vi "HGCalSensorTestingPanel2.vi"() -> ()   [LabVIEW 2015]
uses:
  <vilib>/Utility/file.llb/Write Delimited Spreadsheet (string).vi
panel:
  out "K237 count":u32
  in  "K237 VISA":refnum<visa-resource-name>
  out "XY Graph 2":cluster{"Y":dbl[], "Y":dbl[]}[](graph)
  out "return count 5":u32
  in  "write buffer 2":string
  out "return count 4":u32
  in  "VISA QT7600":refnum<visa-resource-name>
  in  "write buffer":string
  out "VISA out 3":refnum<visa-resource-name>
  out "return count 3":u32
  in  "byte count 2":u32
  out "XY Graph":cluster{"Y":dbl[], "Y":dbl[]}[](graph)
  out "VISA out 2":refnum<visa-resource-name>
  out "return count 2":u32
  out "error out 2":errorcluster
  in  "byte count":u32
  in  "HP":refnum<visa-resource-name>
  out "VISA out":refnum<visa-resource-name>
  out "return count":u32
  in  "Switch":refnum<visa-resource-name>
  in  "Measurement Data":string[][](table)
  in  "OK Button":bool
  in  "Delay (s):":dbl
  in  "Channel:":dbl
  in  "Voltage (V):":dbl
  out "Channel:":dbl format="%#3_6g"
  out "mV(nA)":dbl
  out "pF":dbl
  out "V":dbl
  out "nA":dbl
  # "C"
  # "A"
  # "V"
  # "1M"
  # "1M"
  # "Single Measurement"
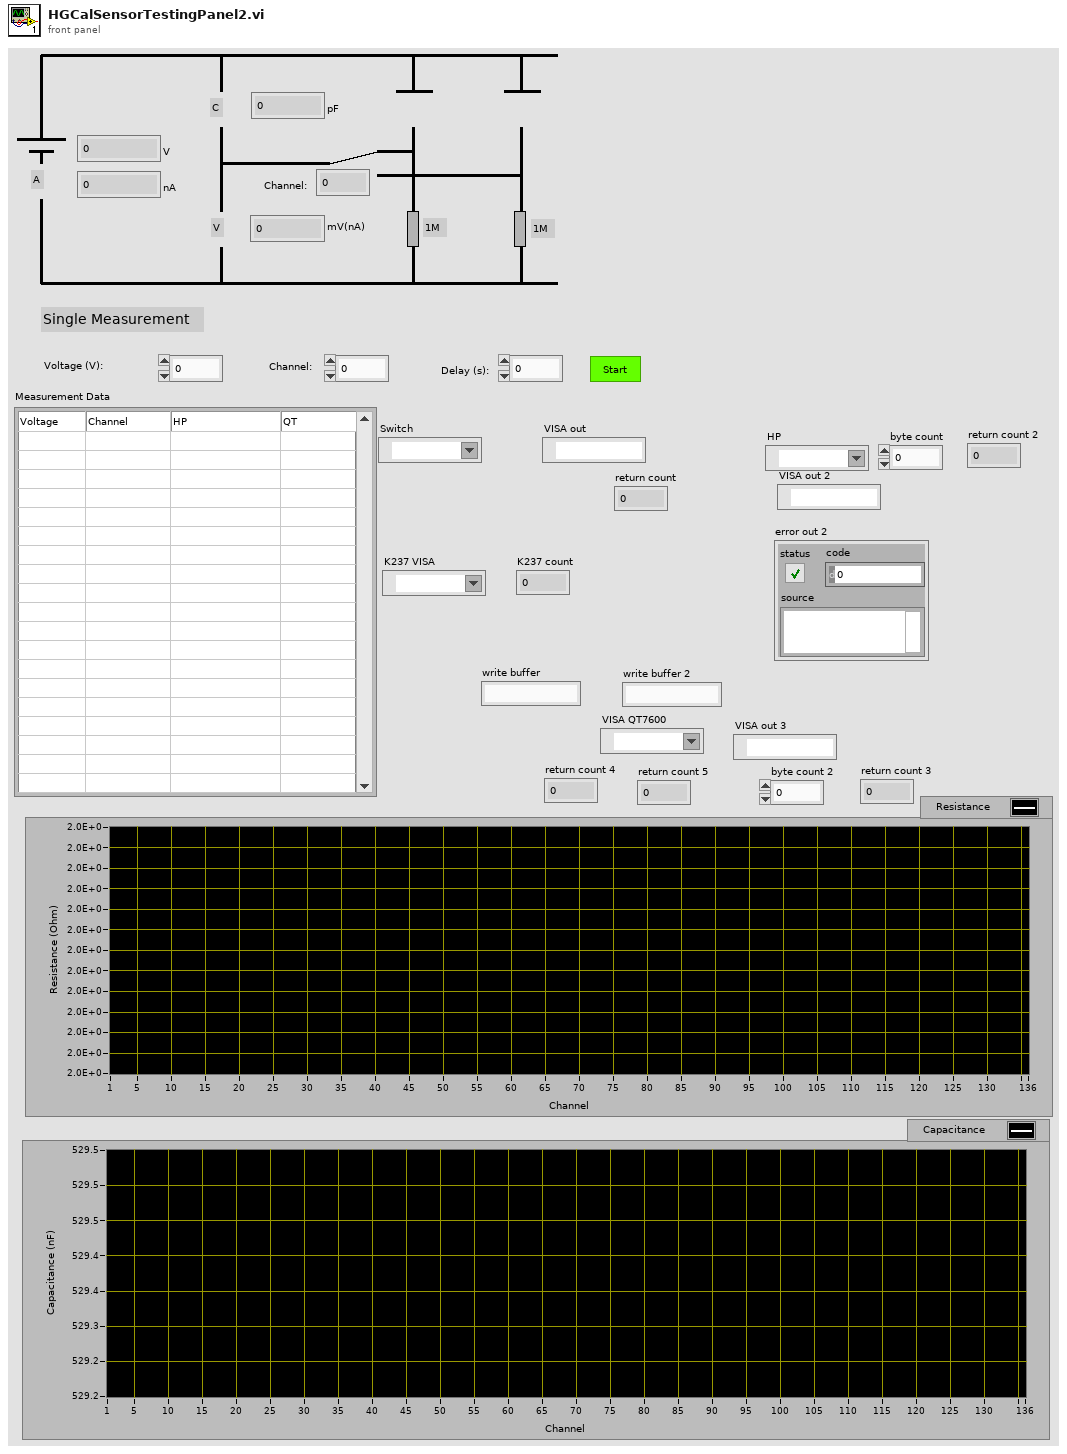
[diagram p1: front panel]
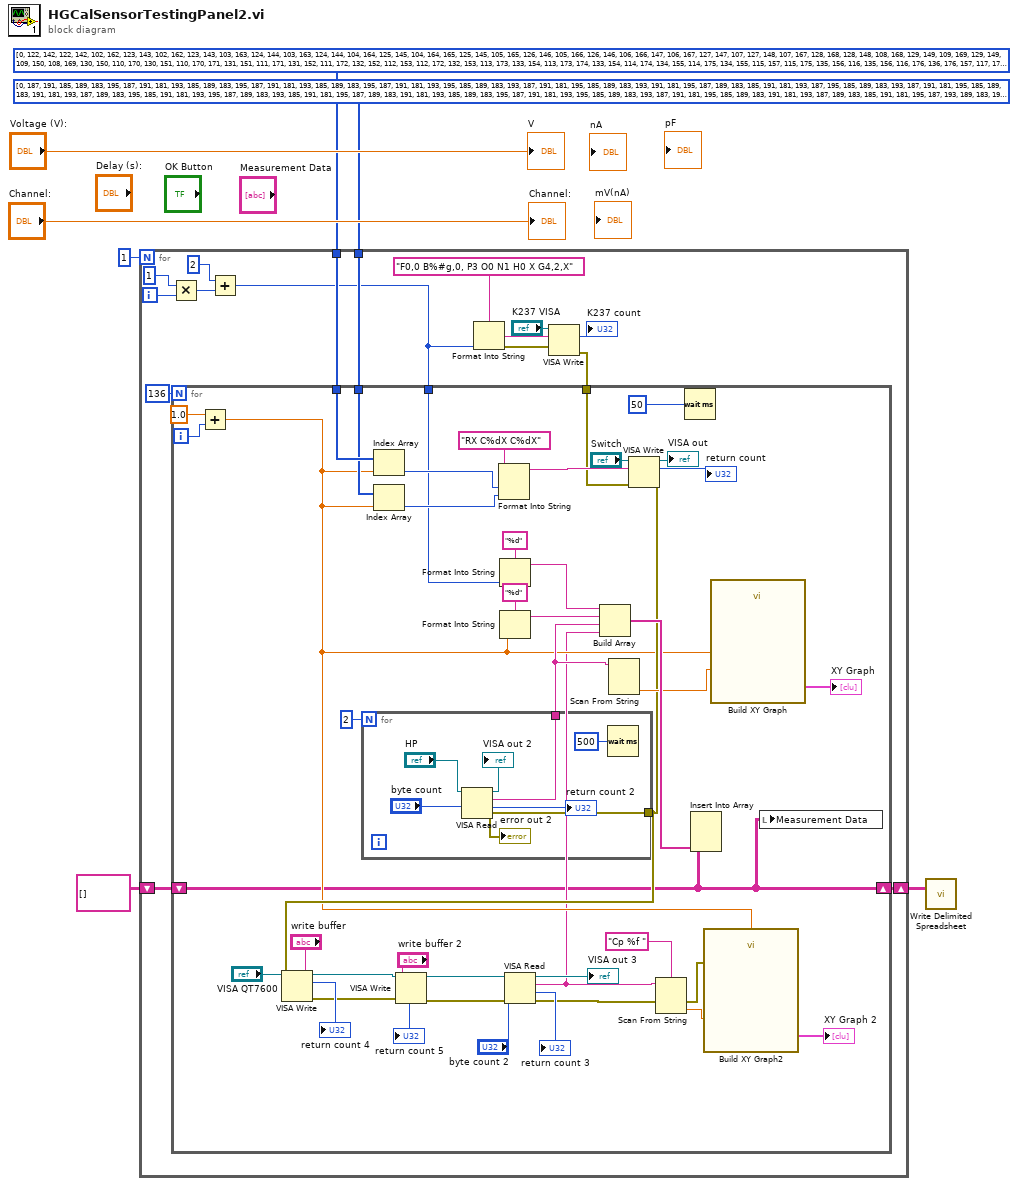
[diagram p0: block diagram]
diagram:
  n1 = for {
    N: 1 -> [_]
    tunnel: i32[] [0, 122, 142, 122, 142, 102, 162, 123, 143, 102, 162, 123, 143, 103, 163, 124, 144, 103, 163, 124, 144, 104, 164, 125, 145, 104, 164, 165, 125, 145, 105, 165, 126, 146, 105, 166, 126, 146, 106, 166, 147, 106, 167, 127, 147, 107, 127, 148, 107, 167, 128, 168, 128, 148, 108, 168, 129, 149, 109, 169, 129, 149, 109, 150, 108, 169, 130, 150, 110, 170, 130, 151, 110, 170, 171, 131, 151, 111, 171, 131, 152, 111, 172, 132, 152, 112, 153, 112, 172, 132, 153, 113, 173, 133, 154, 113, 173, 174, 133, 154, 114, 174, 134, 155, 114, 175, 134, 155, 115, 157, 115, 175, 135, 156, 116, 135, 156, 116, 176, 136, 176, 157, 117, 177, 136, 158, 117, 177, 137, 137, 158, 118, 178, 138, 138, 159, 178] -> [w20]
    tunnel: i32[] [0, 187, 191, 185, 189, 183, 195, 187, 191, 181, 193, 185, 189, 183, 195, 187, 191, 181, 193, 185, 189, 183, 195, 187, 191, 181, 193, 195, 185, 189, 183, 193, 187, 191, 181, 195, 185, 189, 183, 193, 191, 181, 195, 187, 189, 183, 185, 191, 181, 193, 187, 195, 185, 189, 183, 193, 187, 191, 181, 195, 185, 189, 183, 191, 181, 193, 187, 189, 183, 195, 185, 191, 181, 193, 195, 187, 189, 183, 193, 185, 191, 181, 195, 187, 189, 183, 191, 181, 193, 185, 189, 183, 195, 187, 191, 181, 193, 195, 185, 189, 183, 193, 187, 191, 181, 195, 185, 189, 183, 191, 181, 193, 187, 189, 183, 185, 191, 181, 195, 187, 193, 189, 183, 195, 185, 191, 181, 193, 187, 185, 189, 183, 195, 187, 185, 191, 193] -> [w19]
    shift-right: [w21] -> w4
    shift-left: string[][] [] -> [w23]
    i -> [w12]
    n2 = Multiply(x=1 ("y"), y=w12) -> (x*y=w10:i32)
    n3 = Add(x=2 ("y"), y=w10) -> (x+y=w8:i32)
    n4 = Format Into String(format string="F0,0 B%#g,0, P3 O0 N1 H0 X G4,2,X" ("F0,0X B%f,0,X L%f,0X P3X O0X"), w8) -> (resulting string=w14:string, error out=w15:errorcluster)  [unwired: 2 in]
    n5 = VISA Write(VISA resource name="K237 VISA", write buffer=w14, error in (no error)=w15) -> (return count=→"K237 count":u32, error out=w9:errorcluster)  [unwired: 1 out]
    n6 = for {
      N: 136 -> [_]
      shift-right: [w24] -> w21
      shift-left: w23 -> [w24]
      tunnel: w20 -> [w60]
      tunnel: w19 -> [w59]
      tunnel: w9 -> [w26]
      tunnel: w8 -> [w25]
      i -> [w62]
      n7 = Add(x=1.0, y=w62) -> (x+y=w32:dbl)
      n8 = Index Array(array=w60, index=w32) -> (element=w58:i32)
      n9 = Index Array(array=w59, index=w32) -> (element=w57:i32)
      n10 = Format Into String(format string="RX C%dX C%dX", w58, w57) -> (resulting string=w53:string)  [unwired: 2 in, 1 out]
      n11 = Format Into String(format string="%d", w25) -> (resulting string=w67:string)  [unwired: 2 in, 1 out]
      n12 = Format Into String(format string="%d", w32) -> (resulting string=w51:string)  [unwired: 2 in, 1 out]
      n13 = VISA Write(VISA resource name="Switch", write buffer=w53, error in (no error)=w26) -> (VISA resource name out=→"VISA out":refnum<visa-resource-name>, return count=→"return count":u32, error out=w34:errorcluster)
      n14 = VISA Write(VISA resource name="VISA QT7600", write buffer="write buffer", error in (no error)=w34) -> (VISA resource name out=w36:refnum<visa-resource-name>, return count=→"return count 4":u32, error out=w38:errorcluster)
      n15 = for {
        N: 2 -> [_]
        tunnel: [w70] -> w47
        tunnel: w34 -> [w68]
        n16 = VISA Read(VISA resource name="HP", byte count="byte count", error in (no error)=w68) -> (VISA resource name out=→"VISA out 2":refnum<visa-resource-name>, read buffer=w70:string, return count=→"return count 2":u32, error out=→"error out 2":errorcluster)
        n17 = Wait (ms)(milliseconds to wait=u32 500) -> ()  [unwired: 1 out]
      }
      n18 = VISA Write(VISA resource name=w36, write buffer="write buffer 2", error in (no error)=w38) -> (VISA resource name out=w35:refnum<visa-resource-name>, return count=→"return count 5":u32, error out=w37:errorcluster)
      n19 = VISA Read(VISA resource name=w35, byte count="byte count 2", error in (no error)=w37) -> (VISA resource name out=→"VISA out 3":refnum<visa-resource-name>, read buffer=w30:string, return count=→"return count 3":u32, error out=w29:errorcluster)
      n20 = Build Array(w67, w51, w47, w30) -> (w66:string[])
      n21 = Scan From String(input string=w47) -> (output 1=w48:dbl)  [unwired: 4 in, 3 out]
      n22 = Scan From String(format string="Cp %f ", input string=w30, error in=w29) -> (error out=w28:errorcluster, output 1=w31:dbl)  [unwired: 2 in, 2 out]
      n23 = Wait (ms)(milliseconds to wait=u32 50 ("millisecond timer value")) -> ()  [unwired: 1 out]
      n24 = Insert Into Array(array=w24, new element=w66) -> ()  [unwired: 2 in, 1 out]
      n25 = call "Build XY Graph2"("error in (no error)"=w28, "Y Input"=w31, "X Input"=w32) -> ("XY Graph"=→"XY Graph 2":cluster{"X":dbl[], "Y":dbl[]}[])  [unwired: 7 in, 1 out]
      n26 = call "Build XY Graph"("Y Input"=w48, "X Input"=w32) -> ("XY Graph"=→"XY Graph":cluster{"X":dbl[], "Y":dbl[]}[])  [unwired: 8 in, 1 out]
      n27 = local write "Measurement Data"(w24) -> ()
    }
  }
  n28 = call-poly <vilib>:"Write Delimited Spreadsheet.vi"("2D data"=w4) -> ()  [unwired: 13 in, 2 out]
  "V" <- "Voltage (V):"
  "Channel:" <- "Channel:"
